vi "Open And Configure DPI Device.vi"(7 "Pin config":T2(array[cluster])=[{"Pin"="RESET", "Current Limit"=0.01, "Voltage Level"=3.3}, {"Pin"="SCLK", "Current Limit"=0.01, "Voltage Level"=3.3}, {"Pin"="CS", "Current Limit"=0.01, "Voltage Level"=3.3}, {"Pin"="WR", "Current Limit"=0.01, "Voltage Level"=3.3}, {"Pin"="CONVST", "Current Limit"=0.01, "Voltage Level"=0.0}, {"Pin"="REFSEL", "Current Limit"=0.01, "Voltage Level"=3.3}, {"Pin"="STBY", "Current Limit"=0.01, "Voltage Level"=3.3}, {"Pin"="SERPAR", "Current Limit"=0.01, "Voltage Level"=0.0}, {"Pin"="RANGE", "Current Limit"=0.01, "Voltage Level"=0.0}, {"Pin"="OS0", "Current Limit"=0.01, "Voltage Level"=0.0}, {"Pin"="OS1", "Current Limit"=0.01, "Voltage Level"=0.0}, {"Pin"="OS2", "Current Limit"=0.01, "Voltage Level"=0.0}, {"Pin"="RESET", "Current Limit"=0.01, "Voltage Level"=0.0}], 8 "error in (no error)":errorcluster, 9 "TriggerEdge":T1=1800 items=["Rising Edge"=1800, "Falling Edge"=1801], 10 "DPI resource name":string) -> (0 "error out":errorcluster, 2 "DPI Bitfile reference":refnum<k20>, 3 "DPI Session":refnum<k15>)   [LabVIEW 2021]
uses:
  <instrlib>/niDigital/niDigital.llb/niDigital Trigger Digital Edge - Edge.ctl
  <instrlib>/niDigital/niDigital.llb/niDigital Export Signal.ctl
  <instrlib>/niDigital/niDigital.llb/niDigital Conditional Jump Trigger ID.ctl
  <vilib>/Utility/error.llb/Error Cluster From Error Code.vi
  <vilib>/rvi/errors/niLvFpgaAdjustHostInterfaceError.vi
  <instrlib>/niDigital/niDigital.llb/niDigital Load Specifications Levels and Timing (Multiple).vi
  <instrlib>/niDigital/niDigital.llb/niDigital Configure Digital Edge Conditional Jump Trigger.vi
  <instrlib>/niDigital/niDigital.llb/niDigital Create Capture Waveform (Parallel).vi
  <vilib>/rvi/interface/nirviReadWriteControl/nirviReadWriteControl.xnode
  NiFpgaLv.dll
  <vilib>/rvi/interface/Simulation/niFpgaSimulationCallBeginRW.vi
panel:
  in  "dutName":string="AD7606B"
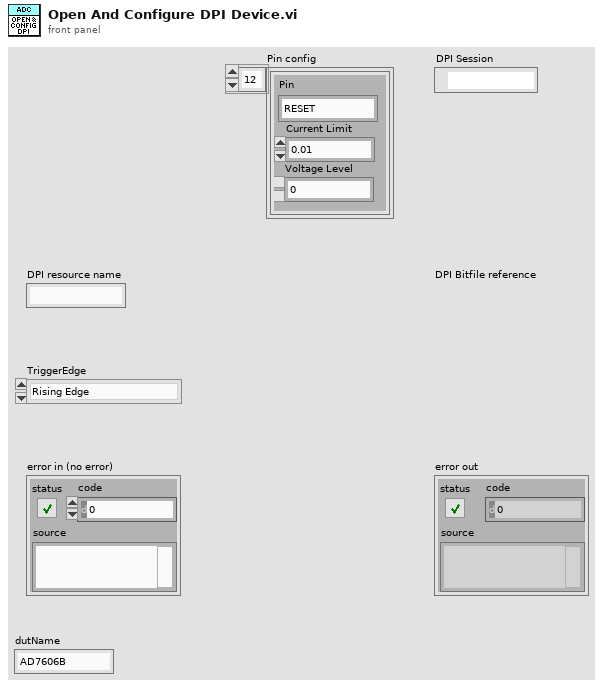
[diagram p1: front panel]
types:
  T1 = typedef "niDigital Trigger Digital Edge - Edge.ctl" = i32
  T2 = cluster{"Pin":string, "Current Limit":dbl, "Voltage Level":dbl}[]
  T3 = typedef "niDigital Conditional Jump Trigger ID.ctl" = string
  T4 = typedef "niDigital Export Signal.ctl" = i32
  T5 = cluster{"high pins":string, "low pins":string, "tristate pins":string}
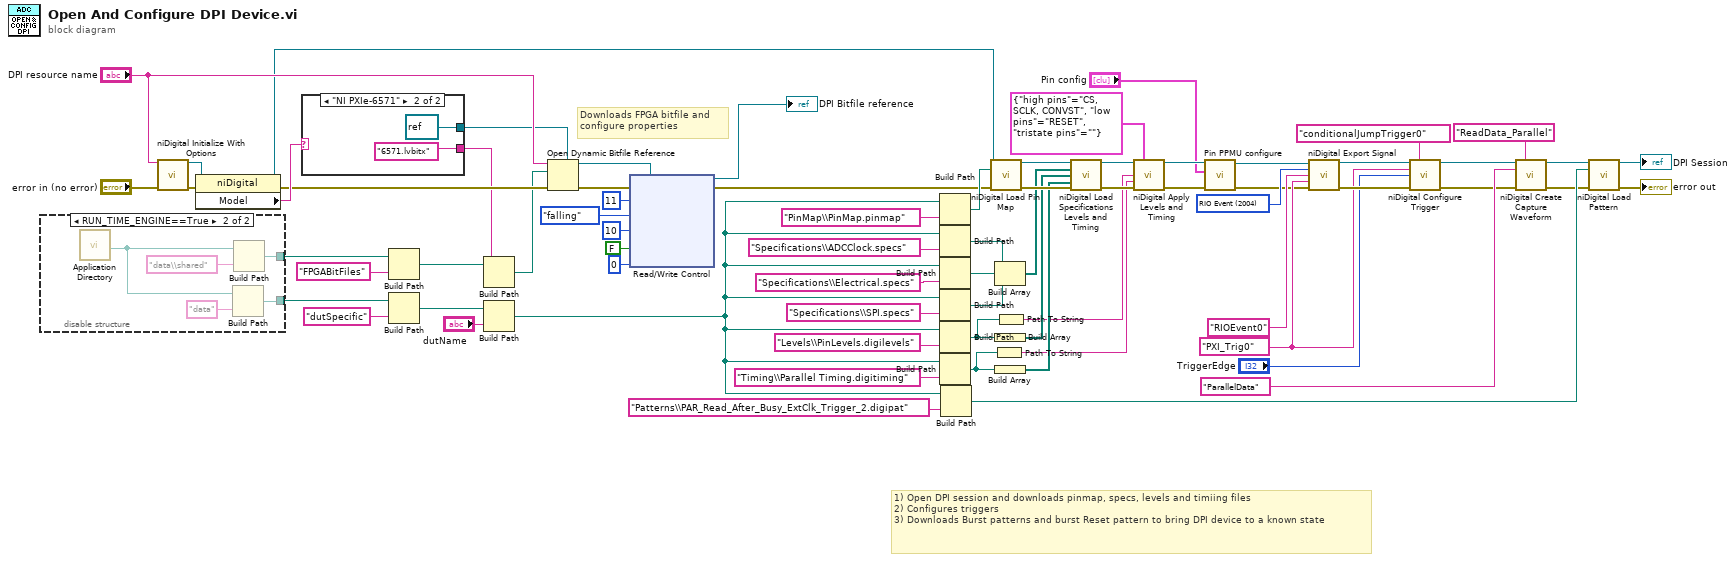
[diagram p0: block diagram]
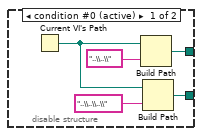
[diagram p2: hidden frame]
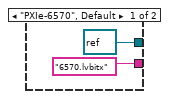
[diagram p3: hidden frame]
diagram:
  w28 = "PXI_Trig0" ("output terminal")
  w31 = T4 2004 items=["Start Trigger"=2000, "Conditional Jump Trigger"=2001, "Pattern Opcode Event"=2002, "RIO Event"=2004] ("signal")
  # "1) Open DPI session and downloads pinmap, specs, levels and timiing files\n2) Configures triggers\n3) Downloads Burst patterns and burst Reset pattern to bring DPI device to a known state"
  # "Downloads FPGA bitfile and\nconfigure properties"
  n1 = disable-structure shown="RUN_TIME_ENGINE==True" {
    disable-tunnel: [w75 w80] -> w2
    disable-tunnel: [w72 w79] -> w1
    frame condition #0 (active) {
      n2 = Current VI's Path() -> (path=w73:path)
      n3 = Build Path(base path=w73, name or relative path="..\\..\\") -> (appended path=w75:path)
      n4 = Build Path(base path=w73, name or relative path="..\\..\\..\\") -> (appended path=w72:path)
    }
    frame condition #1 {
      n5 = call <vilib>:"Application Directory.vi"() -> ("Application Directory"=w78:path)
      n6 = Build Path(base path=w78, name or relative path="data") -> (appended path=w79:path)
      n7 = Build Path(base path=w78, name or relative path="data\\shared") -> (appended path=w80:path)
    }
  }
  n8 = call <instrlib>:"niDigital Initialize With Options.vi"("resource name"="DPI resource name", "error in"="error in (no error)") -> ("instrument handle"=w67:refnum<k15>, "error out"=w66:errorcluster)  [unwired: 12 in]
  n9 = property on="Property Node" class="niDigital"(reference=w67, error in=w66) -> (reference out=w12:refnum<k15>, error out=w68:errorcluster, "Model"=w70:string)
  n10 = case shown="\"NI PXIe-6571\"" w70 {
    tunnel: [refnum<k20> refnum ("Type") refnum<k20> refnum ("Type")] -> w55
    tunnel: ["6570.lvbitx" ("element") "6571.lvbitx" ("element")] -> w65
    frame "PXIe-6570", Default {
    }
    frame "NI PXIe-6571" {
    }
  }
  n11 = Build Path(base path=w2, name or relative path="FPGABitFiles") -> (appended path=w7:path)
  n12 = Build Path(base path=w1, name or relative path="dutSpecific") -> (appended path=w5:path)
  n13 = Build Path(base path=w7, name or relative path=w65) -> (appended path=w64:path)
  n14 = Build Path(base path=w5, name or relative path="dutName") -> (appended path=w3:path)
  n15 = Open Dynamic Bitfile Reference(0:"DPI resource name", 1:w64, 3:w68, 4:w55) -> (5:w57:refnum<k20>, 8:w56:errorcluster)  [unwired: 1 in]
  n16 = xnode "Read/Write Control"("FPGA VI Reference In"=w57, "error in"=w56, "trigger line"=11, "edge"=enum16{"rising", "falling"}."falling", "holdoff time"=u16 10, "active"=FALSE, "delay"=u8 0) -> ("FPGA VI Reference Out"=→"DPI Bitfile reference":refnum<k20>, "error out"=w13:errorcluster)
  n17 = Build Path(base path=w3, name or relative path="PinMap\\PinMap.pinmap" ("element")) -> (appended path=w53:path)
  n18 = Build Path(base path=w3, name or relative path="Specifications\\ADCClock.specs" ("element")) -> (appended path=w44:path)
  n19 = Build Path(base path=w3, name or relative path="Specifications\\Electrical.specs" ("element")) -> (appended path=w45:path)
  n20 = Build Path(base path=w3, name or relative path="Specifications\\SPI.specs" ("element")) -> (appended path=w46:path)
  n21 = Build Path(base path=w3, name or relative path="Levels\\PinLevels.digilevels" ("element")) -> (appended path=w38:path)
  n22 = Build Path(base path=w3, name or relative path="Timing\\Parallel Timing.digitiming" ("element")) -> (appended path=w37:path)
  n23 = Build Path(base path=w3, name or relative path="Patterns\\PAR_Read_After_Busy_ExtClk_Trigger_2.digipat" ("element")) -> (appended path=w22:path)
  n24 = call <instrlib>:"niDigital Load Pin Map.vi"("instrument handle"=w12, "pin map file"=w53, "error in"=w13) -> ("instrument handle out"=w52:refnum<k15>, "error out"=w51:errorcluster)  [unwired: 11 in]
  n25 = Path To String(path=w37) -> (string=w36:string)
  n26 = Build Array(w44, w45, w46) -> (w43:path[])
  n27 = Build Array(w38) -> (w42:path[])
  n28 = Build Array(w37) -> (w41:path[])
  n29 = Path To String(path=w38) -> (string=w35:string)
  n30 = call-poly <instrlib>:"niDigital Load Specifications Levels and Timing.vi"("instrument handle"=w52, "specifications file paths"=w43, "levels file paths"=w42, "timing file paths"=w41, "error in"=w51) -> ("instrument handle out"=w40:refnum<k15>, "error out"=w39:errorcluster)  [unwired: 9 in]
  n31 = call <instrlib>:"niDigital Apply Levels and Timing.vi"("instrument handle"=w40, "initial state"=T5 {"high pins"="CS, SCLK, CONVST", "low pins"="RESET", "tristate pins"=""}, "levels sheet"=w35, "timing sheet"=w36, "error in"=w39) -> ("instrument handle out"=w17:refnum<k15>, "error out"=w15:errorcluster)  [unwired: 9 in]
  n32 = call "Pin PPMU configure.vi"("error in (no error)"=w15, "Pin config"="Pin config", "IVI Refnum in"=w17) -> ("error out"=w14:errorcluster, "IVI Refnum out"=w16:refnum<k15>)  [unwired: 7 in]
  n33 = call <instrlib>:"niDigital Export Signal.vi"("instrument handle"=w16, "signal"=w31, "signal ID"="RIOEvent0" ("element"), "output terminal"=w28, "error in"=w14) -> ("instrument handle out"=w33:refnum<k15>, "error out"=w32:errorcluster)  [unwired: 9 in]
  n34 = call-poly <instrlib>:"niDigital Configure Trigger.vi"("instrument handle"=w33, "trigger ID"=T3 "conditionalJumpTrigger0", "source"=w28, "edge"="TriggerEdge", "error in"=w32) -> ("instrument handle out"=w25:refnum<k15>, "error out"=w24:errorcluster)  [unwired: 9 in]
  n35 = call-poly <instrlib>:"niDigital Create Capture Waveform.vi"("instrument handle"=w25, "waveform name"="ReadData_Parallel" ("pin list"), "pin list"="ParallelData", "error in"=w24) -> ("instrument handle out"=w21:refnum<k15>, "error out"=w20:errorcluster)  [unwired: 10 in]
  n36 = call <instrlib>:"niDigital Load Pattern.vi"("instrument handle"=w21, "pattern file"=w22, "error in"=w20) -> ("instrument handle out"=→"DPI Session":refnum<k15>, "error out"=→"error out":errorcluster)  [unwired: 11 in]
